vi "niDTS BT UTIL Get Standard.vi"(10 "Data Rate":i32=1, 11 "Packet type":T1=enum."DH1") -> (3 "BT Standard":T2 caption="802.11 Standard")   [LabVIEW 2015, in "niDTS BT.lvlib"]
uses:
  niDTS BT.lvlib
  Includes/niDTS BT INC Standard.ctl
  Includes/niDTS BT INC Packet Type.ctl
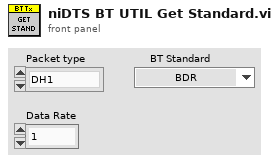
[diagram p1: front panel]
types:
  T1 = typedef "niDTS BT.lvlib/niDTS BT INC Packet Type.ctl" = enum16{"NULL", "POLL", "FHS", "DM1", "DH1", "HV1", "HV2", "HV3", "EV3", "DV", "AUX1", "DM3", "DH3", "EV4", "EV5", "DM5", "DH5", "LE-TP"}
  T2 = typedef "niDTS BT.lvlib/niDTS BT INC Standard.ctl" = enum16{"BDR", "EDR", "LE-TP"}
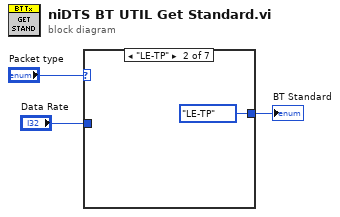
[diagram p0: block diagram]
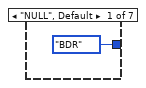
[diagram p2: hidden frame]
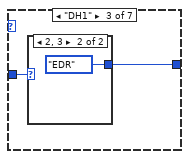
[diagram p3: hidden frame]
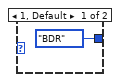
[diagram p4: hidden frame]
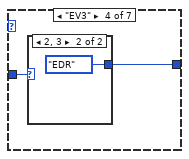
[diagram p5: hidden frame]
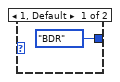
[diagram p6: hidden frame]
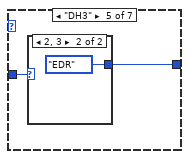
[diagram p7: hidden frame]
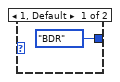
[diagram p8: hidden frame]
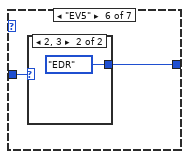
[diagram p9: hidden frame]
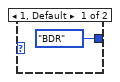
[diagram p10: hidden frame]
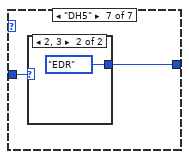
[diagram p11: hidden frame]
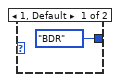
[diagram p12: hidden frame]
diagram:
  n1 = case shown="\"LE-TP\"" "Packet type" {
    tunnel: "Data Rate" -> [_ _ w7 w10 w14 w18 w22]
    tunnel: [niDTS_BT_INC_Standard."BDR" ("BT Standard") niDTS_BT_INC_Standard."LE-TP" ("BT Standard") w6 w11 w15 w19 w23] -> w3
    frame "NULL", Default {
    }
    frame "LE-TP" {
    }
    frame "DH1" {
      n2 = case shown="2, 3" w7 {
        tunnel: [niDTS_BT_INC_Standard."BDR" ("BT Standard") niDTS_BT_INC_Standard."EDR" ("BT Standard")] -> w6
        frame 1, Default {
        }
        frame 2, 3 {
        }
      }
    }
    frame "EV3" {
      n3 = case shown="2, 3" w10 {
        tunnel: [niDTS_BT_INC_Standard."BDR" ("BT Standard") niDTS_BT_INC_Standard."EDR" ("BT Standard")] -> w11
        frame 1, Default {
        }
        frame 2, 3 {
        }
      }
    }
    frame "DH3" {
      n4 = case shown="2, 3" w14 {
        tunnel: [niDTS_BT_INC_Standard."BDR" ("BT Standard") niDTS_BT_INC_Standard."EDR" ("BT Standard")] -> w15
        frame 1, Default {
        }
        frame 2, 3 {
        }
      }
    }
    frame "EV5" {
      n5 = case shown="2, 3" w18 {
        tunnel: [niDTS_BT_INC_Standard."BDR" ("BT Standard") niDTS_BT_INC_Standard."EDR" ("BT Standard")] -> w19
        frame 1, Default {
        }
        frame 2, 3 {
        }
      }
    }
    frame "DH5" {
      n6 = case shown="2, 3" w22 {
        tunnel: [niDTS_BT_INC_Standard."BDR" ("BT Standard") niDTS_BT_INC_Standard."EDR" ("BT Standard")] -> w23
        frame 1, Default {
        }
        frame 2, 3 {
        }
      }
    }
  }
  "BT Standard" <- w3
